vi "Temp - Calibrate.vi"(8 "error in (no error)":errorcluster, 10 "Perform Auto Calibration":bool, 11 "LockinDAQ in":refnum<class "LockinDAQ.lvclass">) -> (0 "error out":errorcluster, 2 "Cal Info":T1(array[cluster]), 3 "LockinDAQ out":refnum<class "LockinDAQ.lvclass">)   [LabVIEW 2016, in "LockinDAQ.lvclass"]
uses:
  LockinDAQ.lvclass
  LockinDAQ.lvclass/LockinDAQ.ctl
  <vilib>/addons/WireFlow/_WF_ProgressBar.llb/WindowBehavior.ctl
  <userlib>/_OpenG.lib/array/array.llb/Remove Duplicates from 1D Array (String)__ogtk.vi
  <vilib>/addons/WireFlow/_WF_ProgressBar.llb/ProgressBar_WireFlow.lvclass
  <resource>/objmgr/daqmx.rc
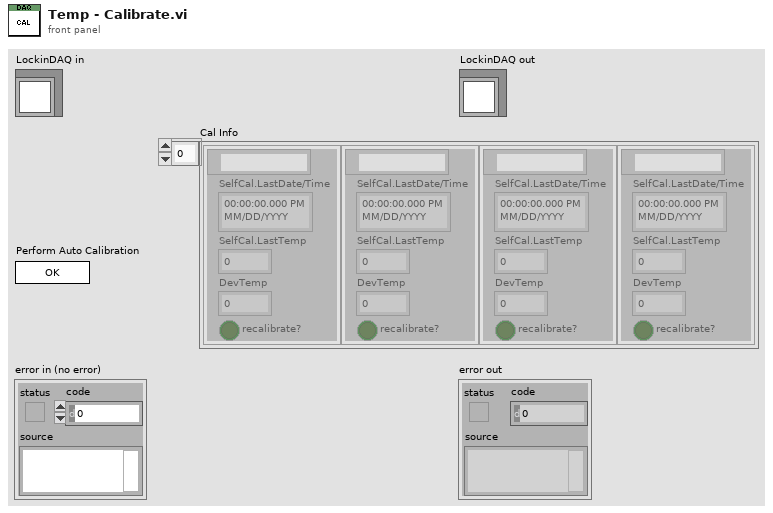
[diagram p1: front panel]
types:
  T1 = cluster{tag, "SelfCal.LastDate/Time":timestamp, "SelfCal.LastTemp":dbl, "DevTemp":dbl, "recalibrate?":bool}[]
  T2 = typedef "ProgressBar_WireFlow.lvclass/WindowBehavior.ctl" = enum16{"No change", "Modal", "Floating"}
  T3 = cluster{"String":string, "SelfCal.LastDate/Time":timestamp, "SelfCal.LastTemp":dbl, "DevTemp":dbl, bool}
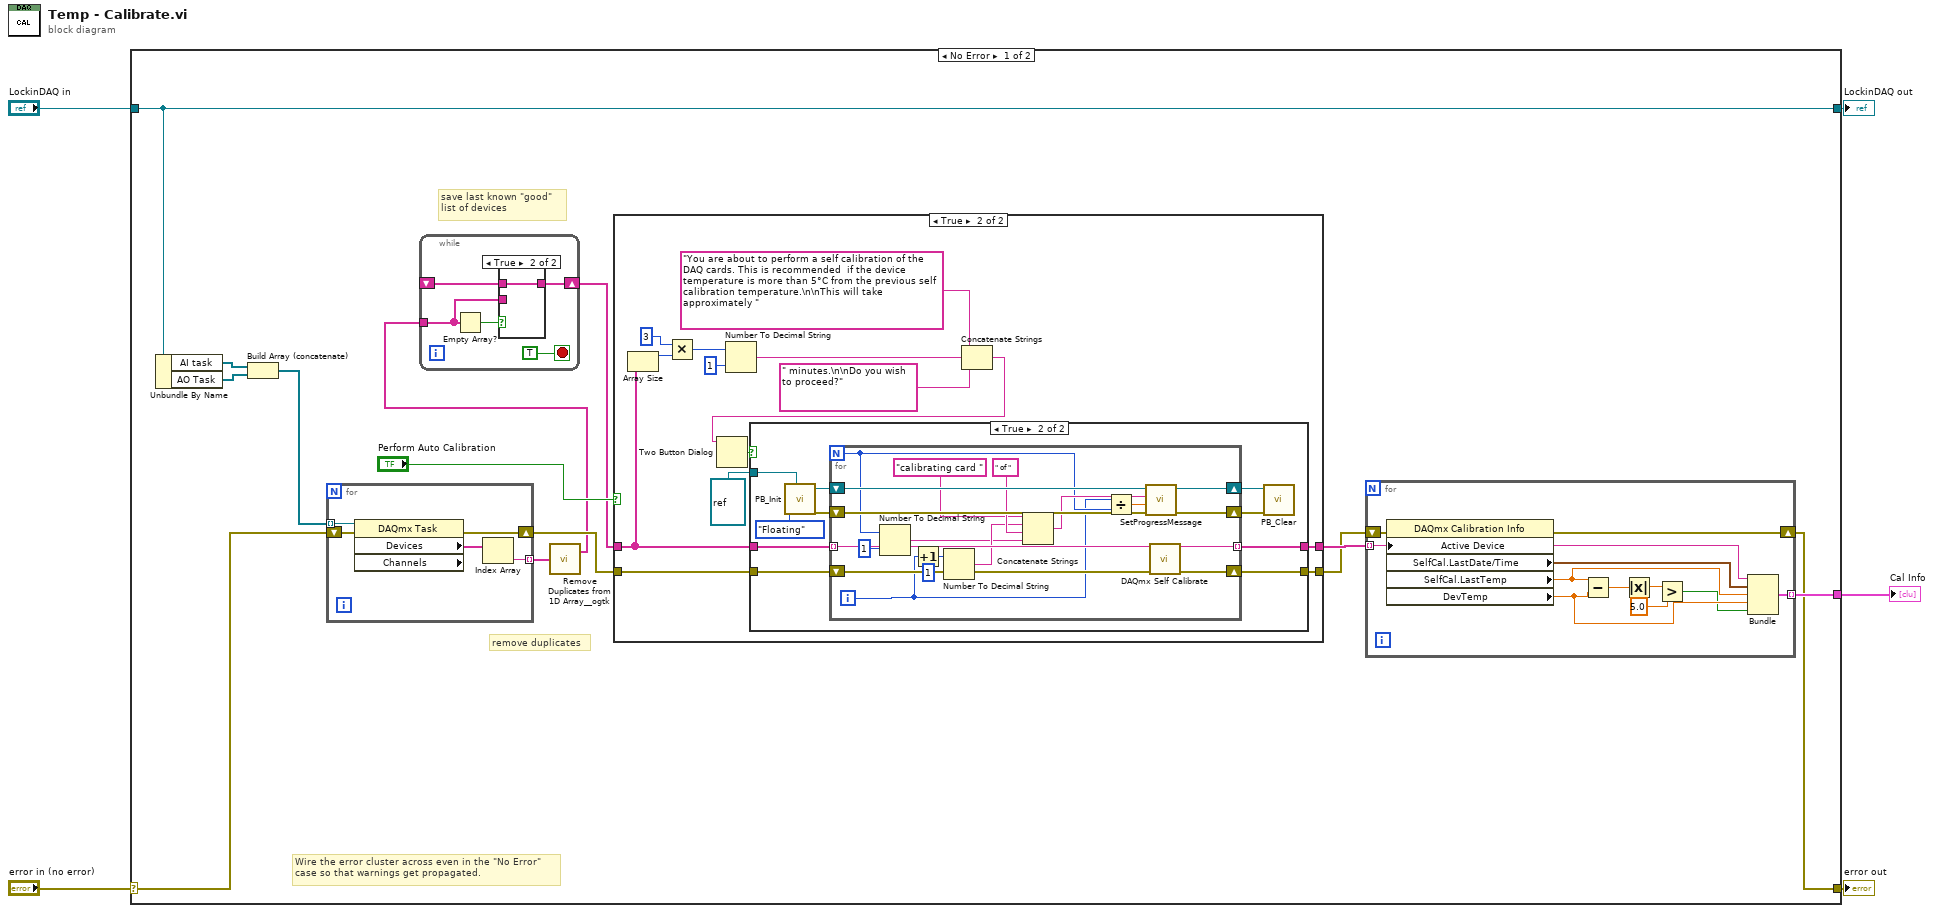
[diagram p0: block diagram]
diagram:
  n1 = case shown="No Error" "error in (no error)" {
    selector: "error in (no error)" -> [w7 w90]
    tunnel: [w6 w90] -> w4
    tunnel: [w12 w89] -> w2
    tunnel: "LockinDAQ in" -> [w12 w89]
    tunnel: [w8 _] -> w1
    frame No Error {
      # "save last known \"good\"\nlist of devices"
      # "remove duplicates"
      # "Wire the error cluster across even in the \"No Error\"\ncase so that warnings get propagated."
      n2 = Unbundle By Name(w12) -> ("AI task"=w11:refnum<k21>[], "AO Task"=w10:refnum<k21>[])
      n3 = Build Array (concatenate)(w11, w10) -> (w9:refnum<k21>[])
      n4 = for {
        tunnel: [w33] -> w19 mode=indexing
        shift-right: [w34] -> w18
        shift-left: w7 -> [w35]
        tunnel: w9 -> [w31] mode=indexing
        n5 = property class="DAQmx Task" props=["Devices", "Channels"](reference=w31, error in=w35) -> (error out=w34:errorcluster, "Devices"=w32:tag[])  [unwired: 2 out]
        n6 = Index Array(array=w32) -> (element=w33:tag)  [unwired: 1 in]
      }
      n7 = call-poly <userlib>:"Remove Duplicates from 1D Array__ogtk.vi"("Input Array"=w19) -> ("Output Array"=w14:string[])  [unwired: 1 out]
      n8 = while {
        shift-right: [w38] -> w13
        shift-left: _ -> [w36]
        tunnel: w14 -> [w37]
        stop <- TRUE stop-if-true
        n9 = Empty Array?(array=w37) -> (empty?=w39:bool)
        n10 = case shown="True" w39 {
          tunnel: [w41 w42] -> w38
          tunnel: w37 -> [w41 _]
          tunnel: w36 -> [_ w42]
          frame False {
          }
          frame True {
          }
        }
      }
      n11 = case shown="True" "Perform Auto Calibration" {
        tunnel: w18 -> [w44 w58]
        tunnel: [w44 w57] -> w16
        tunnel: w13 -> [w43 w55]
        tunnel: [w43 w56] -> w17
        frame False {
        }
        frame True {
          n12 = Array Size(array=w55) -> (size(s)=w54:i32)
          n13 = Multiply(x=3, y=w54) -> (x*y=w46:i32)
          n14 = Number To Decimal String(number=w46, width (-)=i16 1) -> (decimal integer string=w47:string)
          n15 = Concatenate Strings("You are about to perform a self calibration of the DAQ cards. This is recommended  if the device temperature is more than 5°C from the previous self calibration temperature.\n\nThis will take approximately " ("message"), w47, " minutes.\n\nDo you wish to proceed?") -> (w48:string)
          n16 = Two Button Dialog(message=w48) -> (T button?=w49:bool)  [unwired: 2 in]
          n17 = case shown="True" w49 {
            tunnel: w58 -> [w60 w70]
            tunnel: [w60 w69] -> w57
            tunnel: [w59 w68] -> w56
            tunnel: w55 -> [w59 w67]
            tunnel: refnum<vi> refnum ("Progress VI") -> [_ w62]
            frame False {
            }
            frame True {
              n18 = call <vilib>:"PB_Init.vi"("Progress VI"=w62, "Window behavior (No change)"=WindowBehavior."Floating") -> ("error out"=w63:errorcluster, "WF-ProgressBar out"=w64:refnum<class "ProgressBar_WireFlow.lvclass">)  [unwired: 8 in]
              n19 = for {
                N -> [w77]
                shift-right: [w87] -> w69
                shift-left: w70 -> [w88]
                tunnel: w67 -> [w86] mode=indexing
                tunnel: [w86] -> w68 mode=indexing
                shift-right: [w83] -> w66
                shift-left: w64 -> [w84]
                shift-right: [w82] -> w65
                shift-left: w63 -> [w85]
                i -> [w72]
                n20 = Number To Decimal String(number=w77, width (-)=i16 1) -> (decimal integer string=w73:string)
                n21 = Increment(x=w72) -> (x+1=w71:i32)
                n22 = Number To Decimal String(number=w71, width (-)=i16 1) -> (decimal integer string=w75:string)
                n23 = Concatenate Strings("calibrating card ", w75, " of ", w73) -> (w78:string)
                n24 = Divide(x=w72, y=w77) -> (x/y=w79:dbl)
                n25 = call-dynamic "SetProgressMessage.vi"("error in (no error)"=w85, "Progress value (NaN no update)"=w79, "Message"=w78, "WF-ProgressBar in"=w84) -> ("error out"=w82:errorcluster, "WF-ProgressBar out"=w83:refnum<class "ProgressBar_WireFlow.lvclass">)  [unwired: 5 in, 1 out]
                n26 = call <vilib>:"DAQmx Self Calibrate.vi"("device in"=w86, "error in"=w88) -> ("error out"=w87:errorcluster)  [unwired: 13 in]
              }
              n27 = call-dynamic "PB_Clear.vi"("error in (no error)"=w65, "WF-ProgressBar in"=w66) -> ()  [unwired: 8 in, 2 out]
            }
          }
        }
      }
      n28 = for {
        tunnel: [w29] -> w8 mode=indexing
        shift-right: [w30] -> w6
        shift-left: w16 -> [w28]
        tunnel: w17 -> [w20] mode=indexing
        n29 = property class="DAQmx Calibration Info"(error in=w28, "Active Device"=w20) -> (error out=w30:errorcluster, "SelfCal.LastDate/Time"=w24:timestamp, "SelfCal.LastTemp"=w23:dbl, "DevTemp"=w22:dbl)  [unwired: 1 in, 1 out]
        n30 = Subtract(x=w23, y=w22) -> (x-y=w27:dbl)
        n31 = Absolute Value(x=w27) -> (abs(x)=w26:dbl)
        n32 = Greater?(x=w26, y=5.0) -> (0:w21:bool)
        n33 = Bundle("String"=w20, "SelfCal.LastDate/Time"=w24, "SelfCal.LastTemp"=w23, "DevTemp"=w22, w21) -> (w29:T3)  [unwired: 1 in]
      }
    }
    frame Error {
    }
  }
  "error out" <- w4
  "LockinDAQ out" <- w2
  "Cal Info" <- w1
